vi "Configure Wi-Fi.vi"(8 "error in (no error)":errorcluster, 9 "Wi-Fi configuration":T1, 10 "hardware interface index":u16, 11 "PLBB in":refnum<class "PL BlackBox Modbus Client.lvclass">) -> (0 "error out":errorcluster, 3 "PLBB out":refnum<class "PL BlackBox Modbus Client.lvclass">)   [LabVIEW 2015, in "PL BlackBox Modbus Client.lvclass"]
doc: "Configures the Wi-Fi."
uses:
  PL BlackBox Modbus Client.lvclass
  <vilib>/plasmapper/PL Modbus Client/PL Modbus Client.lvclass
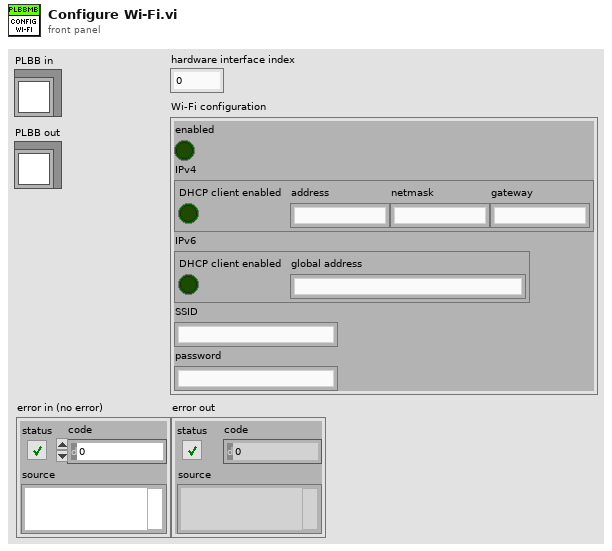
[diagram p1: front panel]
types:
  T1 = cluster{"enabled":bool, "IPv4":cluster{"DHCP client enabled":bool, "address":string, "netmask":string, "gateway":string}, "IPv6":cluster{"DHCP client enabled":bool, "global address":string}, "SSID":string, "password":string}
  T2 = cluster{"DHCP client enabled":bool, "address":string, "netmask":string, "gateway":string}
  T3 = cluster{"DHCP client enabled":bool, "global address":string}
  T4 = cluster{"enabled":bool, "IPv4":cluster{"DHCP client enabled":bool, "address":string, "netmask":string, "gateway":string}, "IPv6":cluster{"DHCP client enabled":bool, "global address":string}}
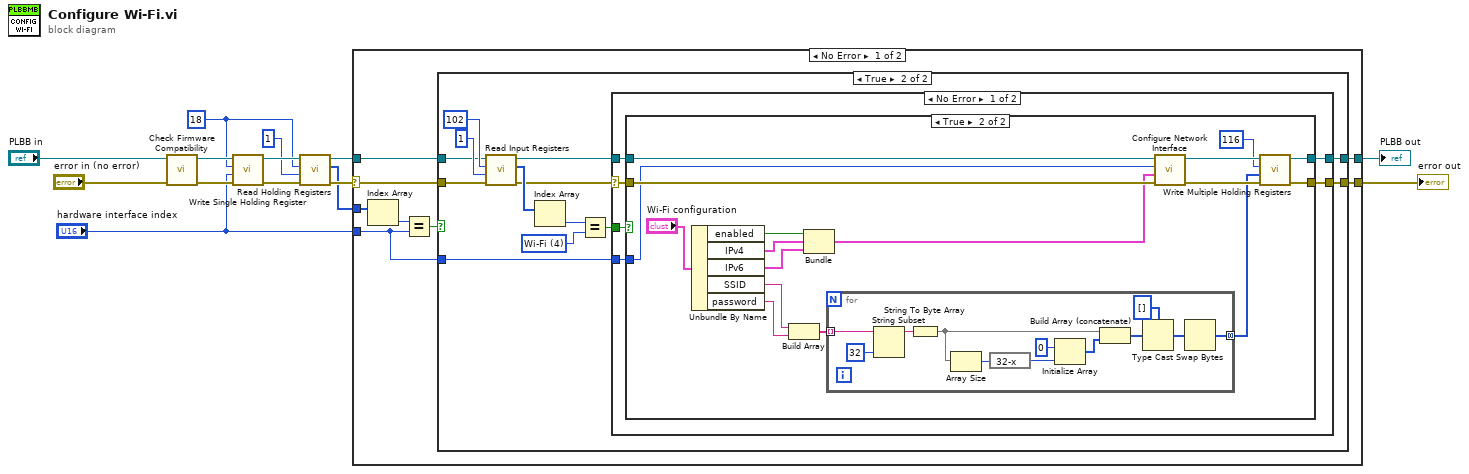
[diagram p0: block diagram]
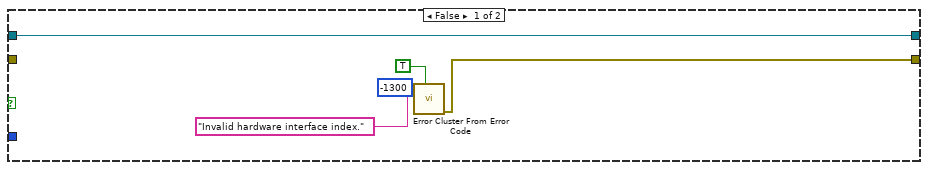
[diagram p2: hidden frame]
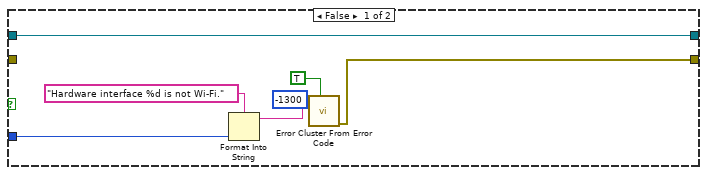
[diagram p3: hidden frame]
diagram:
  w6 = u16 18 ("address")
  n1 = call-dynamic "Check Firmware Compatibility.vi"("error in (no error)"="error in (no error)", "PLBB in"="PLBB in") -> ("error out"=w9:errorcluster, "PLBB out"=w10:refnum<class "PL BlackBox Modbus Client.lvclass">)  [unwired: 8 in]
  n2 = call <vilib>:"Write Single Holding Register.vi"("error in (no error)"=w9, "value"="hardware interface index", "address"=w6, "MODBUS in"=w10) -> ("error out"=w5:errorcluster, "MODBUS out"=w8:refnum<class "PL BlackBox Modbus Client.lvclass">)  [unwired: 6 in]
  n3 = call <vilib>:"Read Holding Registers.vi"("error in (no error)"=w5, "number of holding registers"=u16 1 ("address"), "address"=w6, "MODBUS in"=w8) -> ("error out"=w4:errorcluster, "values"=w2:u16[], "MODBUS out"=w3:refnum<class "PL BlackBox Modbus Client.lvclass">)  [unwired: 5 in]
  n4 = case shown="No Error" w4 {
    selector: w4 -> [w16 w85]
    tunnel: [w22 w85] -> w14
    tunnel: [w21 w86] -> w13
    tunnel: w3 -> [w17 w86]
    tunnel: w2 -> [w20 _]
    tunnel: "hardware interface index" -> [w15 _]
    frame No Error {
      n5 = Index Array(array=w20) -> (element=w19:u16)  [unwired: 1 in]
      n6 = Equal?(x=w19, y=w15) -> (x = y?=w18:bool)
      n7 = case shown="True" w18 {
        tunnel: [w23 w29] -> w22
        tunnel: [w27 w30] -> w21
        tunnel: w17 -> [w27 w38]
        tunnel: w16 -> [_ w37]
        tunnel: w15 -> [_ w28]
        frame False {
          n8 = call <vilib>:"Error Cluster From Error Code.vi"("show call chain? (False)"=TRUE, "error message (\"\")"="Invalid hardware interface index." ("error message (\"\")"), "error code (0)"=-1300) -> ("error out"=w23:errorcluster)  [unwired: 6 in]
        }
        frame True {
          w34 = u16 4 items=["Unknown", "UART", "Network interface", "Ethernet", "Wi-Fi"] ("type")
          n9 = call <vilib>:"Read Input Registers.vi"("error in (no error)"=w37, "number of input registers"=u16 1 ("address"), "address"=u16 102, "MODBUS in"=w38) -> ("error out"=w32:errorcluster, "values"=w36:u16[], "MODBUS out"=w31:refnum<class "PL BlackBox Modbus Client.lvclass">)  [unwired: 5 in]
          n10 = Index Array(array=w36) -> (element=w35:u16)  [unwired: 1 in]
          n11 = Equal?(x=w35, y=w34) -> (x = y?=w33:bool)
          n12 = case shown="No Error" w32 {
            selector: w32 -> [w44 w83]
            tunnel: w33 -> [w46 _]
            tunnel: [w41 w84] -> w30
            tunnel: w31 -> [w45 w84]
            tunnel: [w42 w83] -> w29
            tunnel: w28 -> [w43 _]
            frame No Error {
              n13 = case shown="True" w46 {
                tunnel: w45 -> [w47 w64]
                tunnel: w44 -> [_ w61]
                tunnel: w43 -> [w50 w56]
                tunnel: [w48 w69] -> w42
                tunnel: [w47 w70] -> w41
                frame False {
                  n14 = Format Into String(format string="Hardware interface %d is not Wi-Fi." ("error message (\"\")"), w50) -> (resulting string=w49:string)  [unwired: 2 in, 1 out]
                  n15 = call <vilib>:"Error Cluster From Error Code.vi"("show call chain? (False)"=TRUE, "error message (\"\")"=w49, "error code (0)"=-1300) -> ("error out"=w48:errorcluster)  [unwired: 6 in]
                }
                frame True {
                  n16 = Unbundle By Name("Wi-Fi configuration") -> ("enabled"=w60:bool, "IPv4"=w59:T2, "IPv6"=w58:T3, "SSID"=w67:string, "password"=w66:string)
                  n17 = Build Array(w67, w66) -> (w65:string[])
                  n18 = Bundle("enabled"=w60, "IPv4"=w59, "IPv6"=w58) -> (w55:T4)  [unwired: 1 in]
                  n19 = for {
                    tunnel: w65 -> [w72] mode=indexing
                    tunnel: [w71] -> w57 mode=concatenating
                    n20 = String Subset(string=w72, length (rest)=32 ("length (rest)")) -> (substring=w76:string)  [unwired: 1 in]
                    n21 = String To Byte Array(string=w76) -> (unsigned byte array=w80:u8[])
                    n22 = Array Size(array=w80) -> (size(s)=w74:i32)
                    n23 = expression code="32-x"(w74) -> (w73:i32)
                    n24 = Initialize Array(u8 0, w73) -> (w81:u8[])
                    n25 = Build Array (concatenate)(w80, w81) -> (w77:u8[])
                    n26 = Type Cast(type=u16[] [] ("values"), x=w77) -> (*(type *) &x=w78:u16[])
                    n27 = Swap Bytes(anything=w78) -> (byte swapped=w71:u16[])
                  }
                  n28 = call "Configure Network Interface.vi"("error in (no error)"=w61, "network interface configuration"=w55, "hardware interface index"=w56, "PLBB in"=w64) -> ("error out"=w62:errorcluster, "PLBB out"=w63:refnum<class "PL BlackBox Modbus Client.lvclass">)  [unwired: 6 in]
                  n29 = call <vilib>:"Write Multiple Holding Registers.vi"("error in (no error)"=w62, "values"=w57, "address"=u16 116, "MODBUS in"=w63) -> ("error out"=w69:errorcluster, "MODBUS out"=w70:refnum<class "PL BlackBox Modbus Client.lvclass">)  [unwired: 6 in]
                }
              }
            }
            frame Error {
            }
          }
        }
      }
    }
    frame Error {
    }
  }
  "error out" <- w14
  "PLBB out" <- w13
